vi "readTimingXML.vi"(8 "error in (no error)":errorcluster, 10 "NativeXML in":refnum<class "NativeXML.lvclass">, 11 "PixelflySettings in":refnum<class "PixelflySettings.lvclass">) -> (0 "error out":errorcluster, 2 "NativeXML out":refnum<class "NativeXML.lvclass">, 3 "PixelflySettings out":refnum<class "PixelflySettings.lvclass">)   [LabVIEW 2009, in "Tools.lvlib" / "Settings.lvlib" / "PixelflySettings.lvclass"]
uses:
  PixelflySettings.lvclass
  NativeXML/NativeXML.lvclass
  PixelflySettings.lvclass/PixelflySettings.ctl
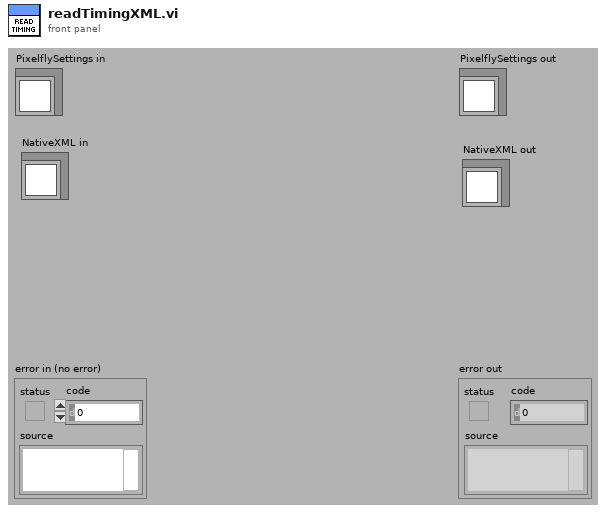
[diagram p1: front panel]
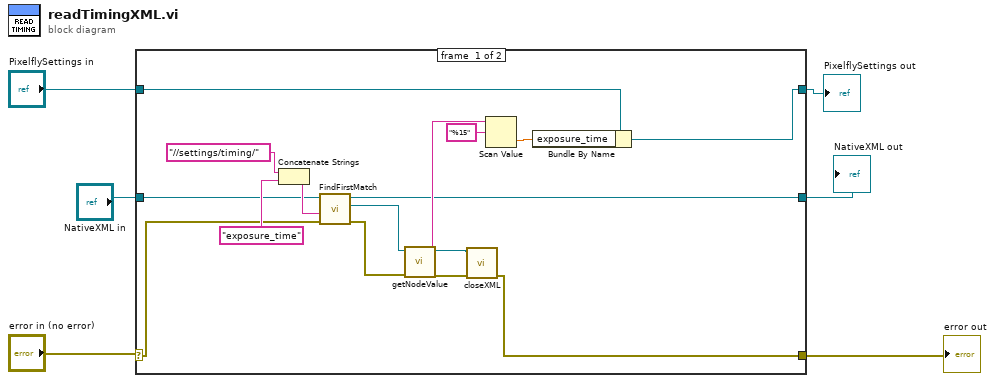
[diagram p0: block diagram]
diagram:
  n1 = case shown="No Error" "error in (no error)" {
    selector: "error in (no error)" -> [w9 w23]
    tunnel: [w15 w23] -> w5
    tunnel: [w21 w24] -> w4
    tunnel: "PixelflySettings in" -> [w22 w24]
    tunnel: "NativeXML in" -> [w7 w25]
    tunnel: [w12 w25] -> w1
    frame #0 {
      n2 = Concatenate Strings("//settings/timing/" ("searchElementIn"), "exposure_time") -> (w8:string)
      n3 = call "FindFirstMatch.vi"("error in (no error)"=w9, "xPath"=w8, "NativeXML in"=w7) -> ("error out"=w10:errorcluster, "NativeXML match"=w11:refnum<class "NativeXML.lvclass">, "NativeXML out"=w12:refnum<class "NativeXML.lvclass">)  [unwired: 6 in]
      n4 = call "getNodeValue.vi"("error in (no error)"=w10, "NativeXML in"=w11) -> ("error out"=w16:errorcluster, "Value"=w20:string, "NativeXML out"=w17:refnum<class "NativeXML.lvclass">)  [unwired: 7 in]
      n5 = call "closeXML.vi"("error in (no error)"=w16, "NativeXML in"=w17) -> ("error out"=w15:errorcluster)  [unwired: 9 in]
      n6 = Scan Value(string=w20, format string="%15") -> (value=w18:dbl)  [unwired: 1 in, 1 out]
      n7 = Bundle By Name(cluster=w22, "exposure_time"=w18) -> (w21:refnum<class "PixelflySettings.lvclass">)
    }
    frame #1 {
    }
  }
  "error out" <- w5
  "PixelflySettings out" <- w4
  "NativeXML out" <- w1
